vi "Reset Progress.vi"(8 "error in (no error)":errorcluster {"code" format="Error %.0f"}, 11 "VIDoc Parser In":refnum<class "VIDoc Parser.lvclass">) -> (0 "error out":errorcluster {"code" format="Error %.0f"}, 3 "VIDoc Parser Out":refnum<class "VIDoc Parser.lvclass">)   [LabVIEW 2023, in "VIDoc Parsing.lvlib" / "VIDoc Parser.lvclass"]
uses:
  VIDoc Parser.lvclass
  VIDoc Parser.lvclass/VIDoc Parser.ctl
  UI Interaction/UI Interaction.lvclass
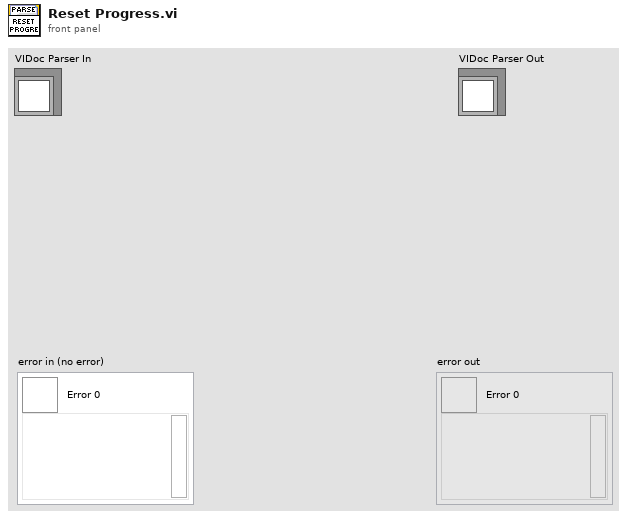
[diagram p1: front panel]
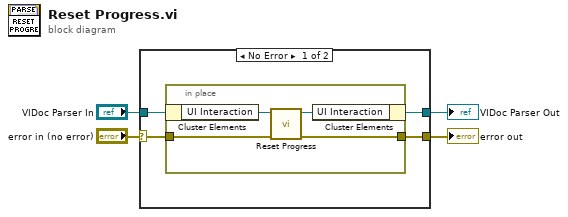
[diagram p0: block diagram]
diagram:
  n1 = case shown="No Error" "error in (no error)" {
    selector: "error in (no error)" -> [w6 w14]
    tunnel: [w5 w14] -> w3
    tunnel: [w8 w13] -> w1
    tunnel: "VIDoc Parser In" -> [w7 w13]
    frame No Error {
      n2 = in-place {
        in-place-border: w6 -> [w10]
        in-place-border: [w9] -> w5
        n3 = in-place-cluster #1(w7) -> ("UI Interaction"=w12:refnum<class "UI Interaction.lvclass">)
        n4 = call "Reset Progress.vi"("error in (no error)"=w10, "UI Interaction in"=w12) -> ("error out"=w9:errorcluster, "UI Interaction out"=w11:refnum<class "UI Interaction.lvclass">)  [unwired: 8 in]
        n5 = in-place-cluster #1("UI Interaction"=w11) -> (w8:refnum<class "VIDoc Parser.lvclass">)
      }
    }
    frame Error {
    }
  }
  "error out" <- w3
  "VIDoc Parser Out" <- w1
